vi "datasource connection.vi"   [LabVIEW 2020]
uses:
  Nominal Client/Nominal Client.lvclass/Nominal Client.ctl
  464d25eb-2538-4162-9245-1f37caa868aa.vi
  Nominal Client/private_data.set.vi
  <vilib>/Utility/file.llb/Application Directory.vi
  <vilib>/Utility/error.llb/Error Cluster From Error Code.vi
  <vilib>/addons/_JKI.lib/REST Client/classes/REST Client/Create REST Client.vi
  Nominal Client/Nominal Client.lvclass
  <vilib>/addons/_JKI.lib/REST Client/classes/REST Client/REST Client.lvclass
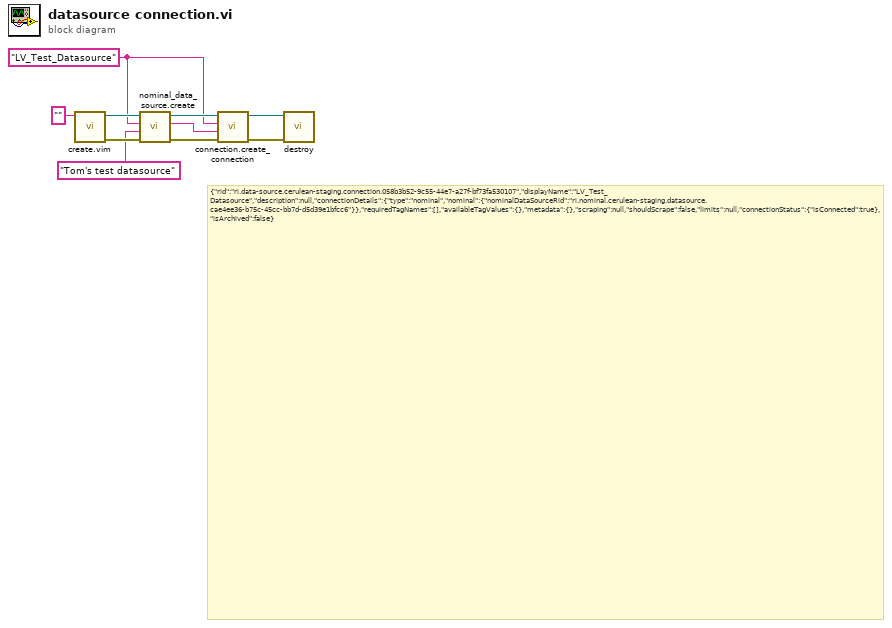
[diagram p0: block diagram]
diagram:
  w2 = "LV_Test_Datasource" ("ID")
  # "{\"rid\":\"ri.data-source.cerulean-staging.connection.058b3b52-9c55-44e7-a27f-bf73fa530107\",\"displayName\":\"LV_Test_Datasource\",\"description\":null,\"connectionDetails\":{\"type\":\"nominal\",\"nominal\":{\"nominalDataSourceRid\":\"ri.nominal.cerulean-staging.datasource.cae4ee36-b75c-45cc-bb7d-d5d39e1bfcc6\"}},\"requiredTagNames\":[],\"availableTagValues\":{},\"metadata\":{},\"scraping\":null,\"shouldScrape\":false,\"limits\":null,\"connectionStatus\":{\"isConnected\":true},\"isArchived\":false}"
  n1 = call "create.vim"("API Token (string or path)"="") -> ("error out"=w3:errorcluster, "Nominal Client"=w7:refnum<class "Nominal Client.lvclass">)  [unwired: 9 in]
  n2 = call "nominal_data_source.create.vi"("error in"=w3, "Description"="Tom's test datasource", "ID"=w2, "Nominal Client in"=w7) -> ("error out"=w4:errorcluster, "rid"=w5:string, "Nominal Client out"=w6:refnum<class "Nominal Client.lvclass">)  [unwired: 3 in, 2 out]
  n3 = call "connection.create_connection.vi"("error in"=w4, "nominalDataSourceRid"=w5, "name"=w2, "Nominal Client in"=w6) -> ("error out"=w9:errorcluster, "Nominal Client out"=w10:refnum<class "Nominal Client.lvclass">)  [unwired: 5 in, 1 out]
  n4 = call "destroy.vi"("error in"=w9, "Nominal Client"=w10) -> ()  [unwired: 9 in, 1 out]
